vi "max.vi"() -> ()   [LabVIEW 2024]
panel:
  in  "x 3":dbl
  out "In Range?":bool
  in  "Numeric 2":dbl
  out "Numeric":i32
  out "x-y*floor(x/y)":dbl
  in  "x 2":dbl
  out "min(x,y)":dbl
  out "max(x,y)":dbl
  in  "y":dbl
  in  "x":dbl
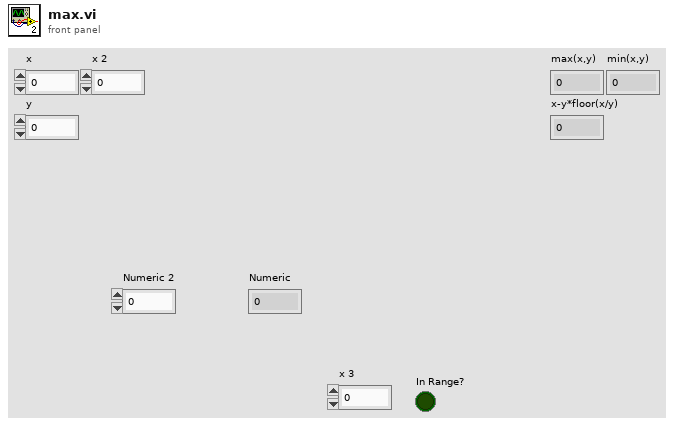
[diagram p1: front panel]
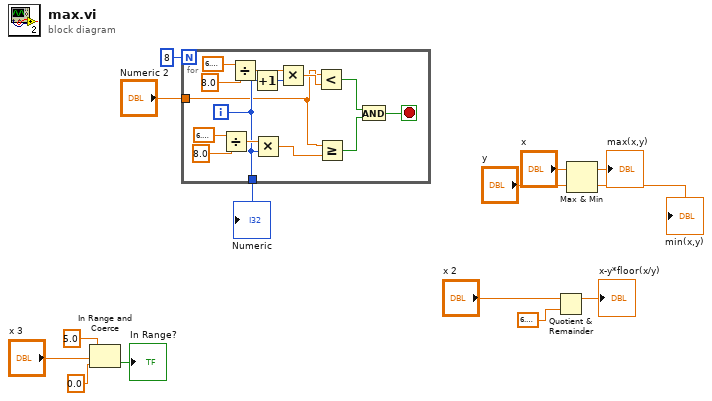
[diagram p0: block diagram]
diagram:
  n1 = In Range and Coerce(upper limit=5.0, x="x 3", lower limit=0.0) -> (In Range?=→"In Range?":bool)  [unwired: 1 out]
  n2 = for {
    N: 8 -> [_]
    tunnel: "Numeric 2" -> [w16]
    tunnel: [w18] -> w6
    i -> [w18]
    stop <- w19 stop-if-true
    n3 = Divide(x=6.283185307179586, y=8.0) -> (x/y=w26:dbl)
    n4 = Divide(x=6.283185307179586, y=8.0) -> (x/y=w23:dbl)
    n5 = Increment(x=w18) -> (x+1=w22:i32)
    n6 = Multiply(x=w26, y=w18) -> (x*y=w15:dbl)
    n7 = Multiply(x=w23, y=w22) -> (x*y=w17:dbl)
    n8 = Less?(x=w16, y=w17) -> (x < y?=w21:bool)
    n9 = Greater Or Equal?(x=w16, y=w15) -> (x >= y?=w20:bool)
    n10 = And(x=w21, y=w20) -> (x .and. y?=w19:bool)
  }
  "Numeric" <- w6
  n11 = Quotient & Remainder(x="x 2", y=6.283185307179586) -> (x-y*floor(x/y)=→"x-y*floor(x/y)":dbl)  [unwired: 1 out]
  n12 = Max & Min(x="x", y="y") -> (max(x,y)=→"max(x,y)":dbl, min(x,y)=→"min(x,y)":dbl)
